vi "TestCloneAPI.vi"() -> ()   [LabVIEW 2014, in "FGenModule.lvlib"]
uses:
  FGenModule.lvlib
  FGenPlugins/MyPluginBaseClass/TypeDef/OperateModeParams.ctl
  FGenPlugins/MyPluginBaseClass/TypeDef/OutputEnableParams.ctl
  FGenPlugins/MyPluginBaseClass/TypeDef/OutputModeParams.ctl
  FGenPlugins/MyPluginBaseClass/TypeDef/RefClkSourceParams.ctl
  FGenPlugins/MyPluginBaseClass/TypeDef/ChannelNameParams.ctl
  FGenPlugins/MyPluginBaseClass/TypeDef/ConfigStdWaveformParams.ctl
  FGenPlugins/MyPluginBaseClass/TypeDef/ClrArbWfrmParams.ctl
  FGenPlugins/MyPluginBaseClass/TypeDef/CreateArbWfrmParams.ctl
  FGenPlugins/MyPluginBaseClass/TypeDef/ConfigArbWfrmParams.ctl
  FGenPlugins/MyPluginBaseClass/TypeDef/ConfigArbWfrmSRatParams.ctl
  FGenPlugins/MyPluginBaseClass/TypeDef/TriggerParams.ctl
  FGenPlugins/MyPluginBaseClass/TypeDef/ChannelParams.ctl
  FGenPlugins/MyPluginBaseClass/TypeDef/ChannelParamElement.ctl
  <userlib>/NIST/ModuleAdminLib/ModuleAdmin/ModuleAdmin.lvclass/ModuleAdmin.ctl
  <userlib>/NIST/ModuleAdminLib/ModuleAdmin/ModuleAdmin.lvclass
  FGenPlugins/MyPluginBaseClass/TypeDef/PluginParams.ctl
  PublicAPI/Arguments/Broadcasts/clDidInit.ctl
  PublicAPI/Arguments/Requests/clStopArgument.ctl
  <userlib>/NIST/ModuleAdminLib/ModuleAdmin/Accessors/Read CloneRegRef.vi
  <userlib>/NIST/ModuleAdminLib/CloneRegistration/CloneRegistration.lvclass
  FGenPlugins/MyPluginBaseClass/NISTFGenPluginsBase.lvclass
panel:
  in  "btnGetTimestamp":bool
  out "Timestamp":timestamp format="%^<%.3X\n%x>T"
  in  "btnConfigDlg":bool
  out "error out":errorcluster
  in  "btnWriteChannel":bool
  in  "btnReadChannel":bool
  in  "ChannelParams":T1 {"eOutputMode" items=["Function", "Arbitrary", "Sequence"]; "eOperateMode" items=["Continuous", "Burst"]}
  in  "btnGetDefaults":bool
  in  "Plugin Type":u16(ring) items=["Keysight 335XX", "none", "HIL FGen", "NI Dynamic 2", "NI Dyn3 FGen", "NI PXI 6733"]
  in  "btnListVISA":bool
  in  "btnSetTrigger":bool
  in  "TriggerParams":T3={"eTrigger"=0, "eEdge"=10280, "sSource"="/PXI1Slot7/PFI1"} {"eEdge" items=["Rising"=10280, "Falling"=10171]; "eTrigger" items=["None", "Digital", "Analog"]}
  in  "ConfigArbWfrmSRatParams":T4
  in  "btnConfigArbWfrmSRat":bool
  in  "ArbWfrmConfig":T5
  in  "btnConfigArbWfrm":bool
  in  "CreateArbWfrmParams":T6={"sName"="1", "iSize"=8, "dData"=[1.0, 1.0, 2.0, 2.5, 2.5, 1.8, 1.8, 1.9, 2.7, 2.9, 1.2], "sWfrmHandle"="ARB1"}
  in  "btnCreateArbWfrm":bool
  in  "ClrArbWfrmParams":T7
  in  "btnClearArbWfrm":bool
  in  "ConfigStdWaveformParams":T8={"sName"="1", "eWaveform"=0, "dAmplitude"=1.0, "dDcOffset"=0.0, "dFrequency"=10.0, "dStartPhase"=0.0, "dSampleRate"=4800.0, "dNumSamples"=4800.0} {"eWaveform" items=["Sine"=0, "Square"=1, "Ramp"=2, "Noise"=3, "DC"=4, "Triangle"=5, "Pulse"=6, "Sinc"=11, "D-Lorentz"=12, "Gaussian"=13, "Expo Fall"=14, "Expo Rise"=15, "Haversine"=16]}
  in  "btnSetStdWaveform":bool
  in  "btnInitialize":bool
  in  "btnReset":bool
  in  "btnAbortGeneration":bool
  out "Channel Name":string
  in  "ChannelNameParams":T9
  in  "RefClkSourceParams":T10 {"eRefClk" items=["Internal", "External", "RTSI"]}
  in  "OutputModeParams":T11 {"eOutputMode" items=["Function", "Arbitrary", "Sequence"]}
  in  "btnInitiateGeneration":bool
  in  "btnChannelNameRequest":bool
  in  "btnSetRefClkSource":bool
  in  "btnSetOutputMode":bool
  in  "OutputEnableParams":T12
  in  "btnSetOutputEnable":bool
  in  "btnSetOperateMode":bool
  in  "OperateModeParams":T13 {"eOperateMode" items=["Continuous", "Burst"]}
  in  "btnLoadPlugin":bool
  out "Path":path
  in  "btnRequestINIPath":bool
  in  "btnRemove":bool
  out "Status Log":string
  out "Active Modules (Array)":string[](array[string])
  in  "btnAdd":bool
  in  "btnStop":bool
  in  "Select Module":i32(ring)=-1 caption="Select Module to send Request" items=["All"=-1]
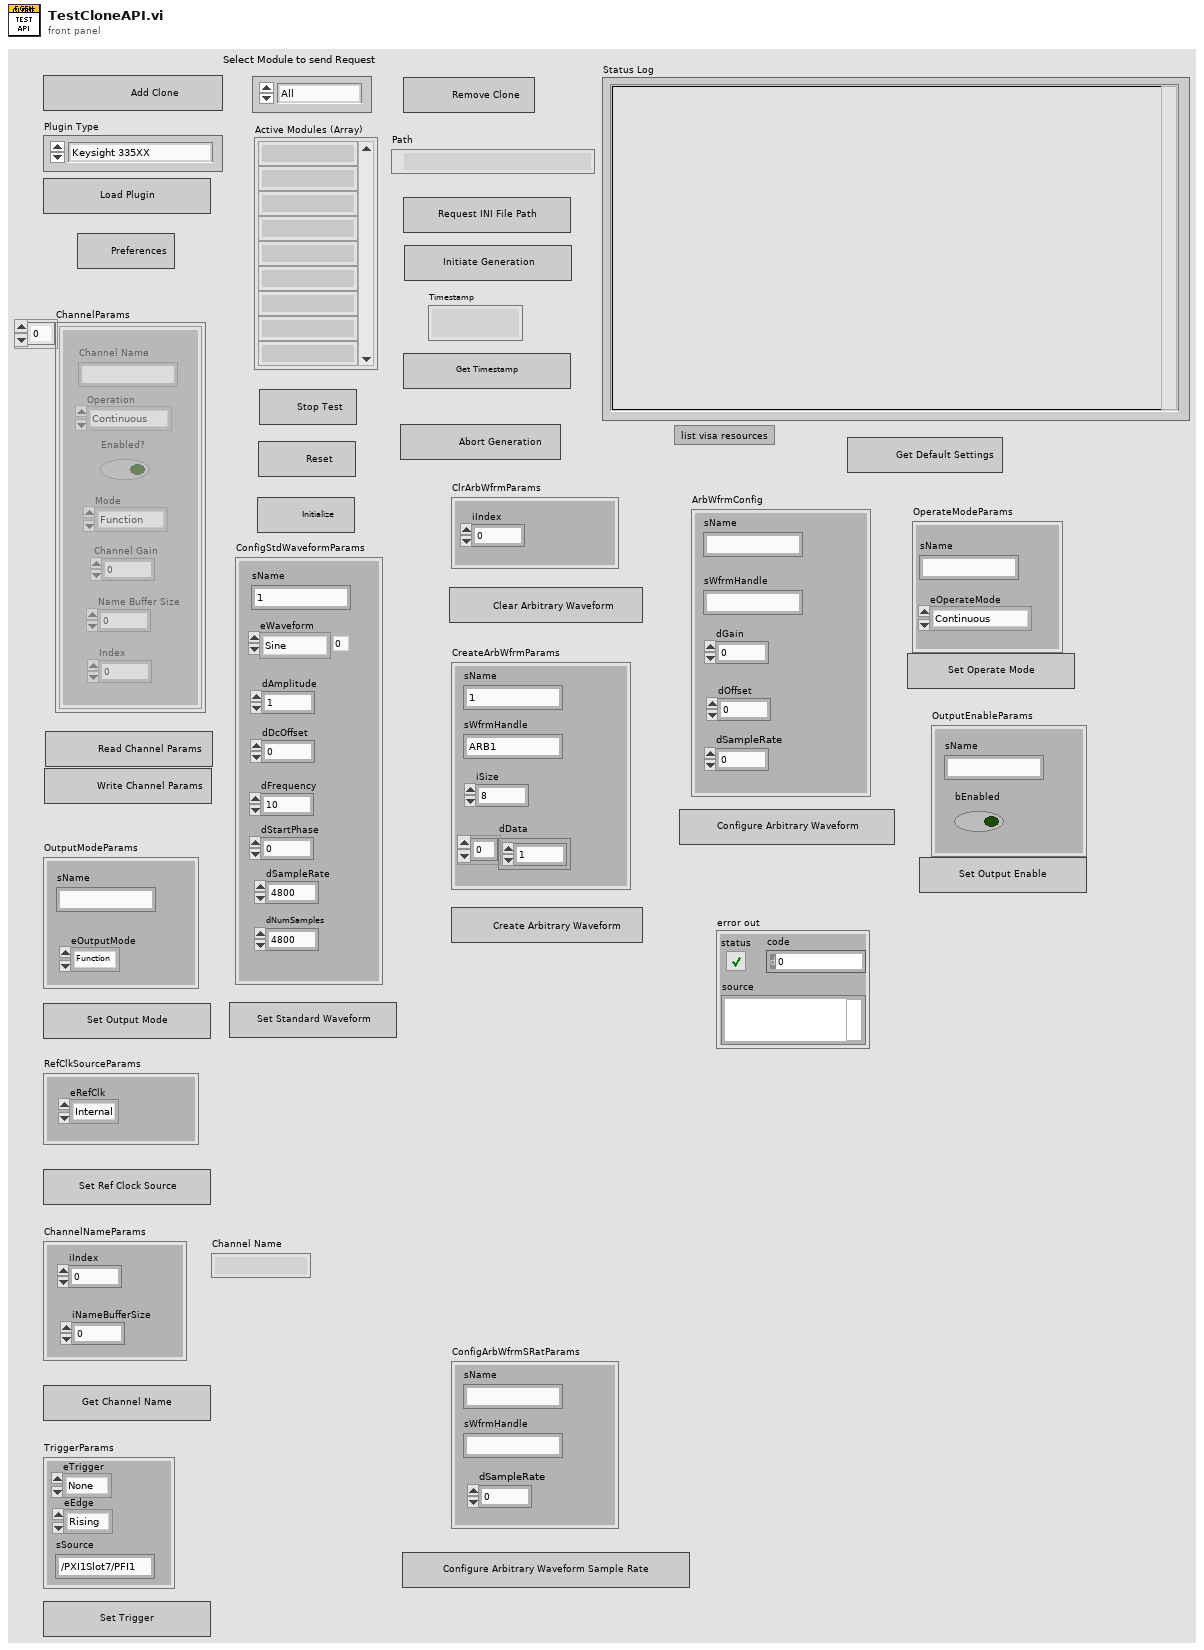
[diagram p1: front panel]
types:
  T1 = typedef "FGenPlugins.lvlib/NISTFGenPluginsBase.lvclass/ChannelParams.ctl" = T2[]
  T2 = typedef "FGenPlugins.lvlib/NISTFGenPluginsBase.lvclass/ChannelParamElement.ctl" = cluster{"sName":string, "eOperateMode":u16, "bEnabled":bool, "eOutputMode":u16, "iIndex":i32, "iNameBufferSize":i32, "fGain":dbl}
  T3 = typedef "FGenPlugins.lvlib/NISTFGenPluginsBase.lvclass/TriggerParams.ctl" = cluster{"eTrigger":u16, "eEdge":u16, "sSource":string}
  T4 = typedef "FGenPlugins.lvlib/NISTFGenPluginsBase.lvclass/ConfigArbWfrmSRatParams.ctl" = cluster{"sName":string, "dSampleRate":dbl, "sWfrmHandle":string}
  T5 = typedef "FGenPlugins.lvlib/NISTFGenPluginsBase.lvclass/ConfigArbWfrmParams.ctl" = cluster{"sName":string, "dGain":dbl, "sWfrmHandle":string, "dOffset":dbl, "dSampleRate":dbl}
  T6 = typedef "FGenPlugins.lvlib/NISTFGenPluginsBase.lvclass/CreateArbWfrmParams.ctl" = cluster{"sName":string, "iSize":i32, "dData":dbl[], "sWfrmHandle":string}
  T7 = typedef "FGenPlugins.lvlib/NISTFGenPluginsBase.lvclass/ClrArbWfrmParams.ctl" = cluster{"iIndex":i32}
  T8 = typedef "FGenPlugins.lvlib/NISTFGenPluginsBase.lvclass/ConfigStdWaveformParams.ctl" = cluster{"sName":string, "eWaveform":u16, "dAmplitude":dbl, "dDcOffset":dbl, "dFrequency":dbl, "dStartPhase":dbl, "dSampleRate":dbl, "dNumSamples":dbl}
  T9 = typedef "FGenPlugins.lvlib/NISTFGenPluginsBase.lvclass/ChannelNameParams.ctl" = cluster{"iIndex":i32, "iNameBufferSize":i32}
  T10 = typedef "FGenPlugins.lvlib/NISTFGenPluginsBase.lvclass/RefClkSourceParams.ctl" = cluster{"eRefClk":u16}
  T11 = typedef "FGenPlugins.lvlib/NISTFGenPluginsBase.lvclass/OutputModeParams.ctl" = cluster{"sName":string, "eOutputMode":u16}
  T12 = typedef "FGenPlugins.lvlib/NISTFGenPluginsBase.lvclass/OutputEnableParams.ctl" = cluster{"sName":string, "bEnabled":bool}
  T13 = typedef "FGenPlugins.lvlib/NISTFGenPluginsBase.lvclass/OperateModeParams.ctl" = cluster{"sName":string, "eOperateMode":u16}
  T14 = typedef "FGenModule.lvlib/clBroadcastEvents.ctl" = cluster{"DidInit":refnum<user-event>, "StatusUpdate":refnum<user-event>, "ErrorReport":refnum<user-event>, "DidStop":refnum<user-event>, "PathToINI":refnum<user-event>, "ChannelName":refnum<user-event>, "ArbWfrmConfig":refnum<user-event>, "ChannelParams":refnum<user-event>, "Timestamp":refnum<user-event>}
  T15 = typedef "FGenPlugins.lvlib/NISTFGenPluginsBase.lvclass/PluginParams.ctl" = cluster{"Path to Plugin INI":path}
  T16 = typedef "FGenModule.lvlib/clDidInit.ctl" = cluster{"Init?":bool, "ModuleAdmin":refnum<class "ModuleAdmin.lvclass">}
  T17 = typedef "FGenModule.lvlib/clStopArgument.ctl" = cluster{"Exit via Stop Module Req?":bool, "Wait for Module to stop?":bool, "ModuleAdmin":refnum<class "ModuleAdmin.lvclass">}
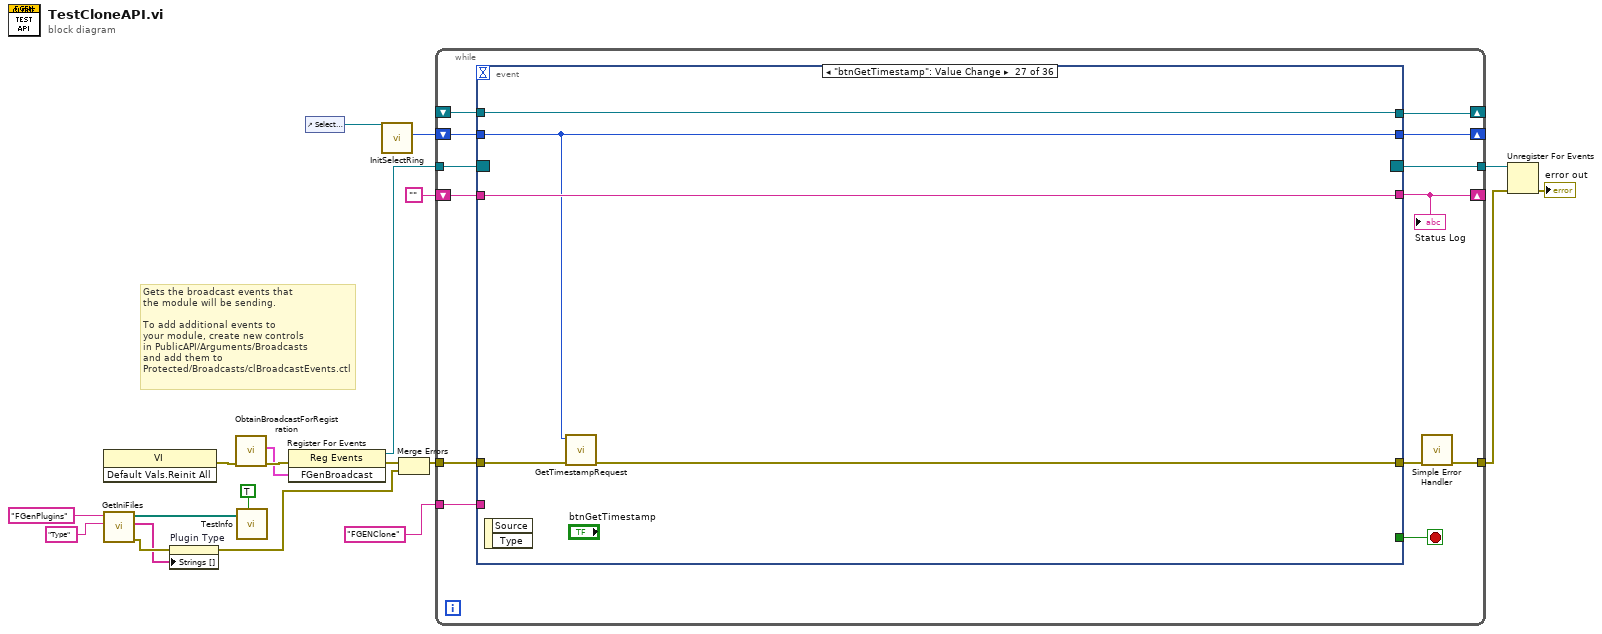
[diagram p0: block diagram]
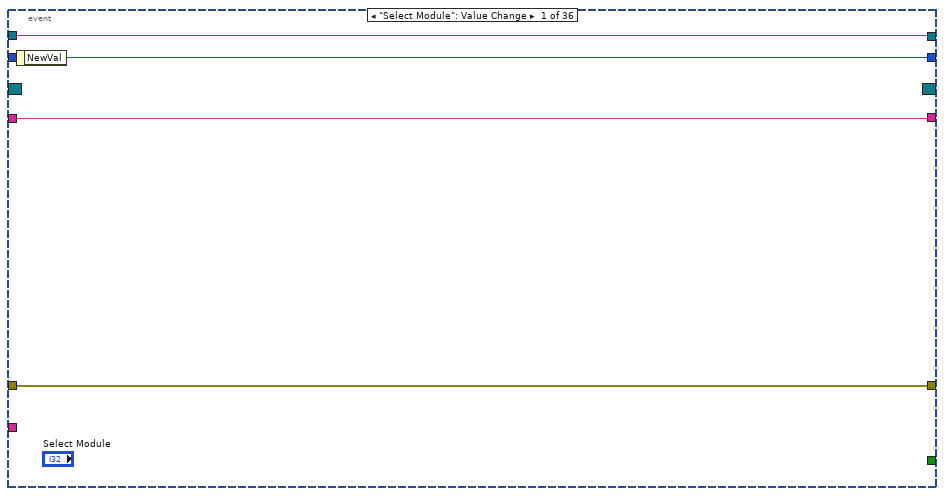
[diagram p2: hidden frame]
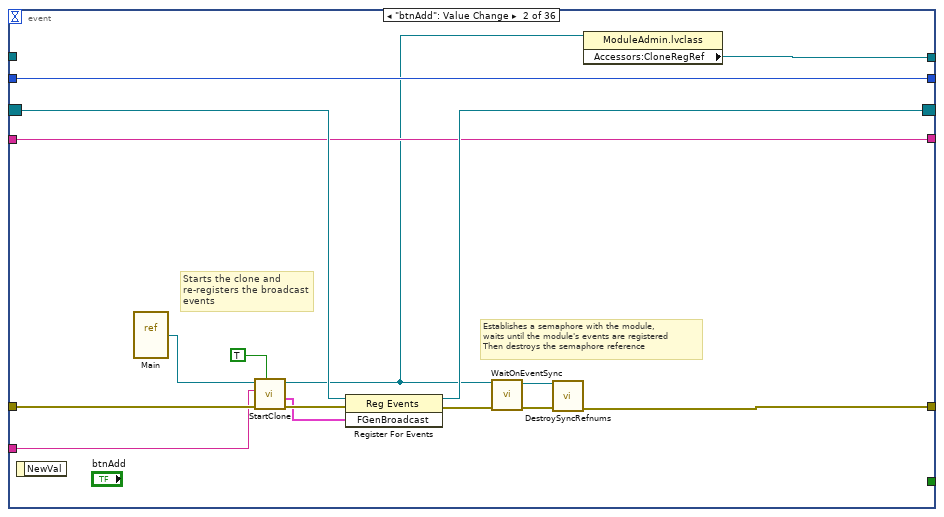
[diagram p3: hidden frame]
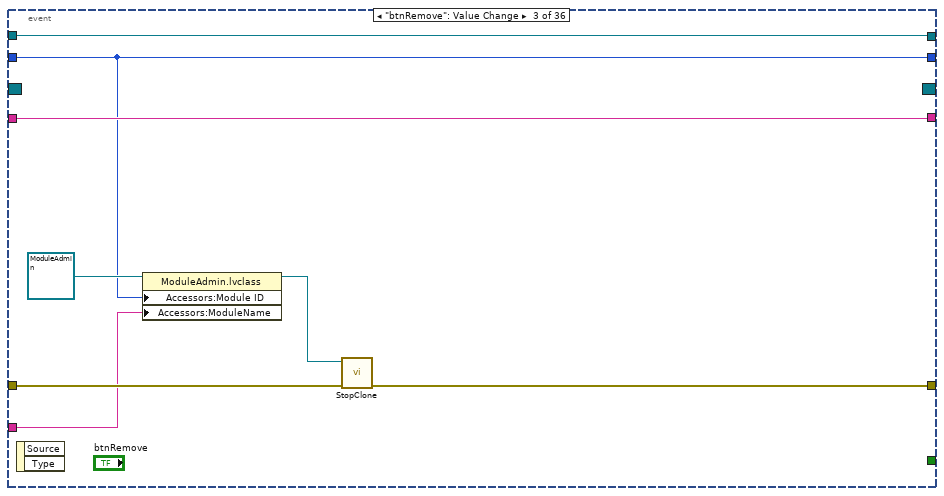
[diagram p4: hidden frame]
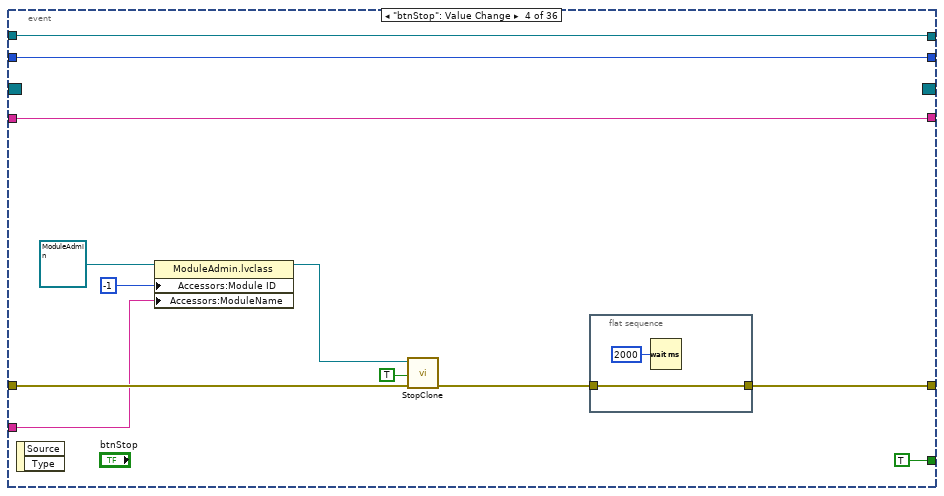
[diagram p5: hidden frame]
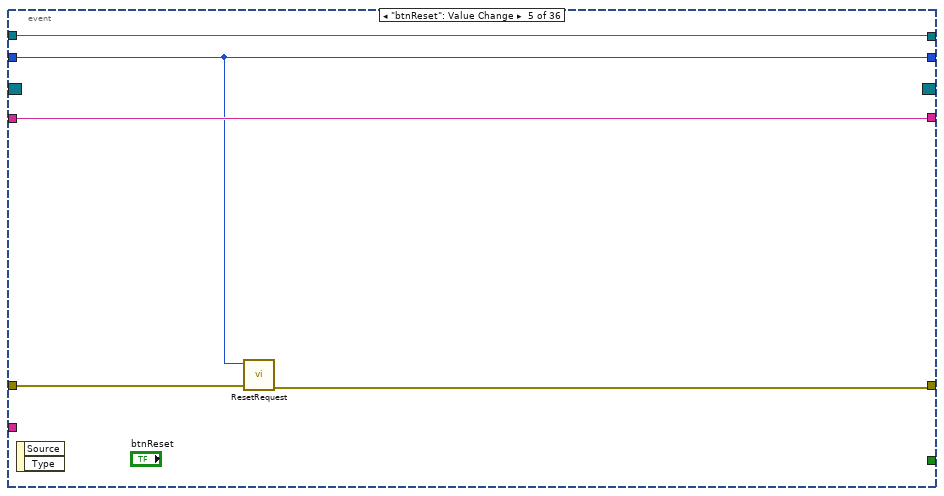
[diagram p6: hidden frame]
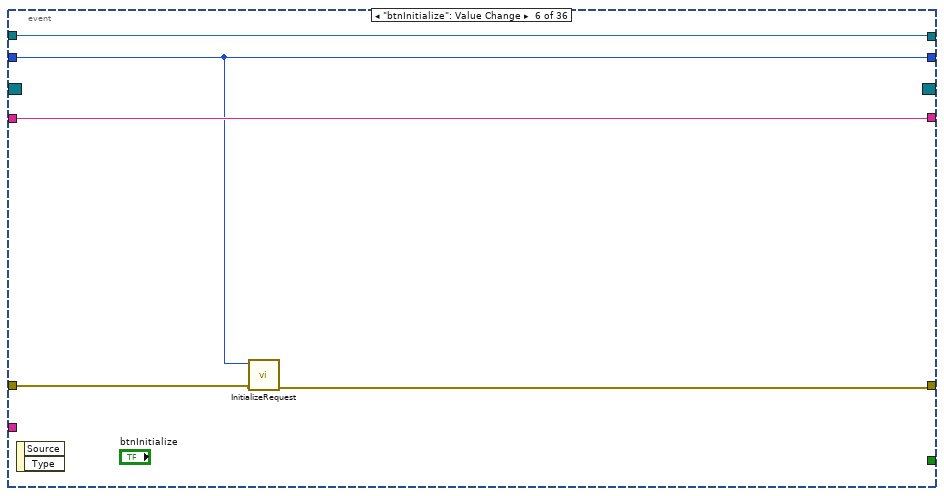
[diagram p7: hidden frame]
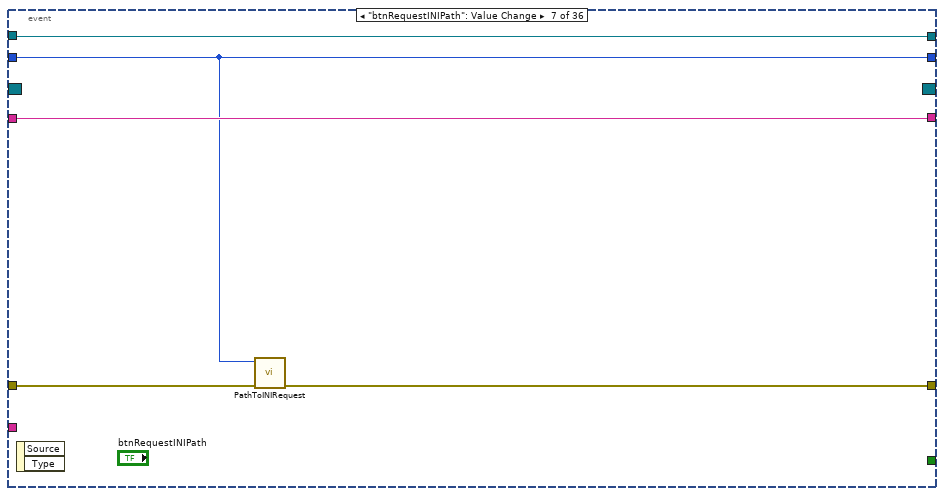
[diagram p8: hidden frame]
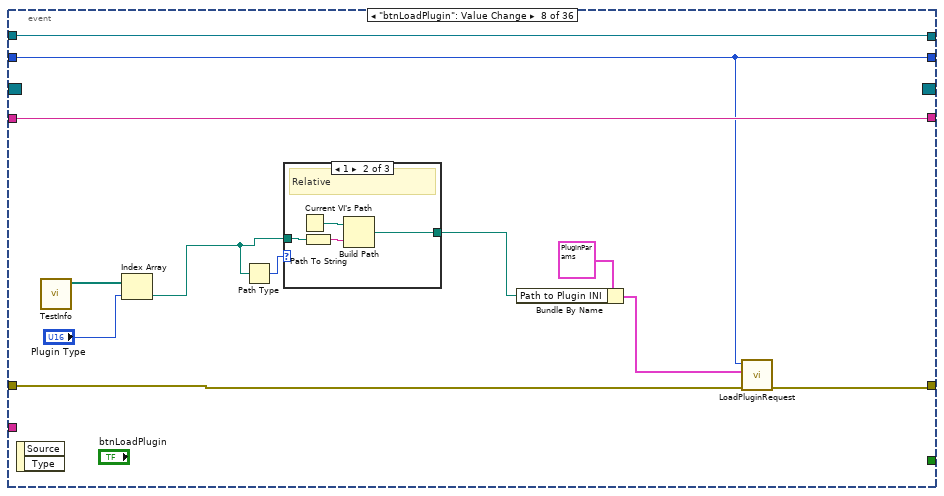
[diagram p9: hidden frame]
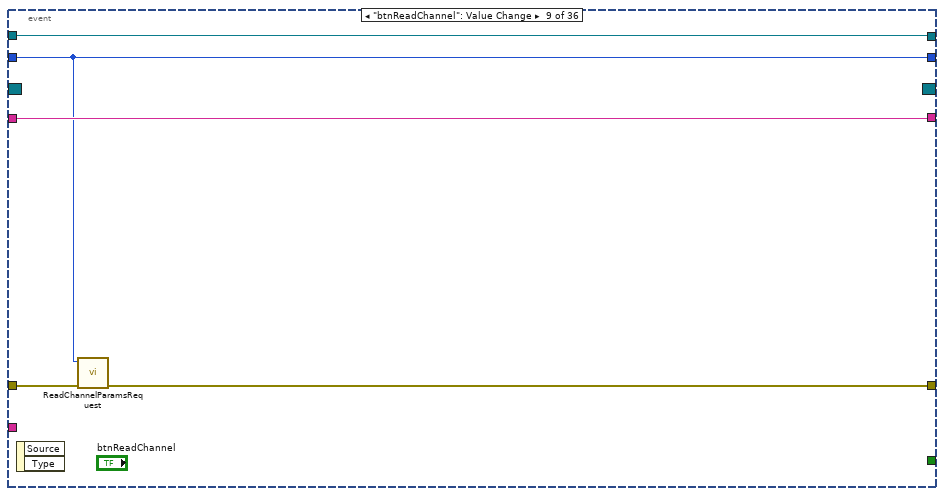
[diagram p12: hidden frame]
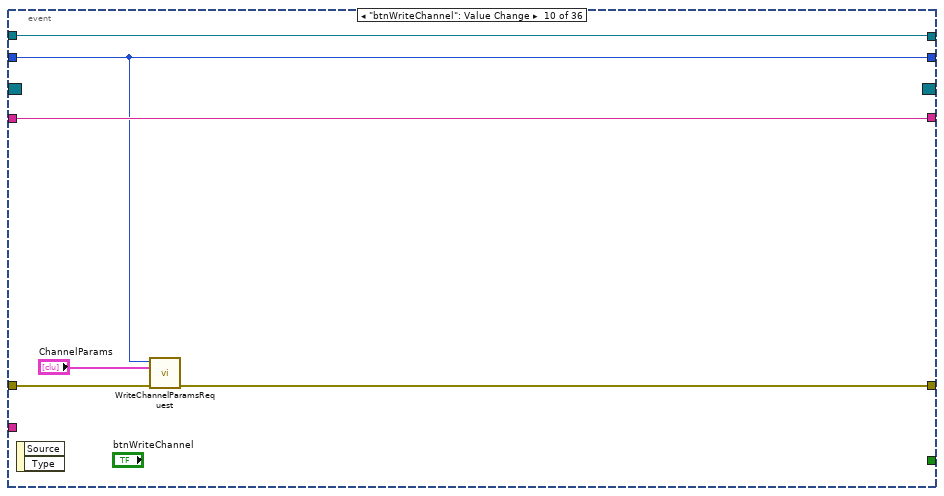
[diagram p13: hidden frame]
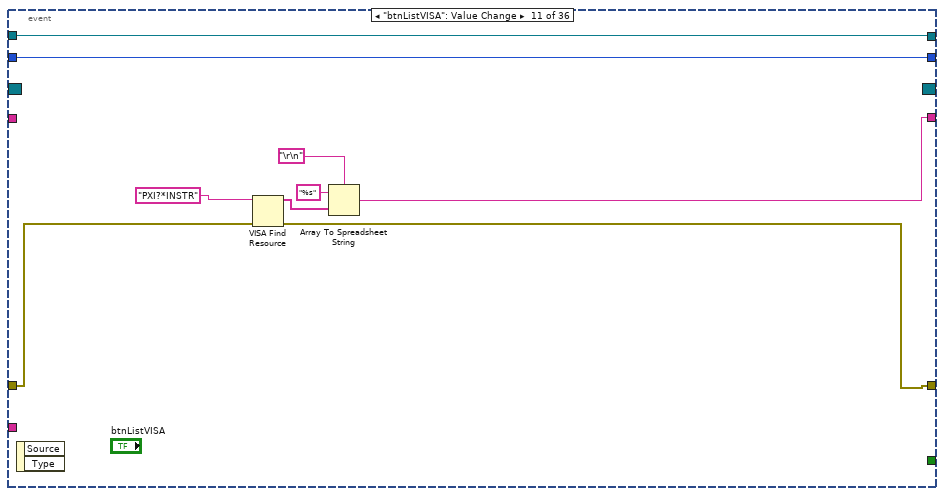
[diagram p14: hidden frame]
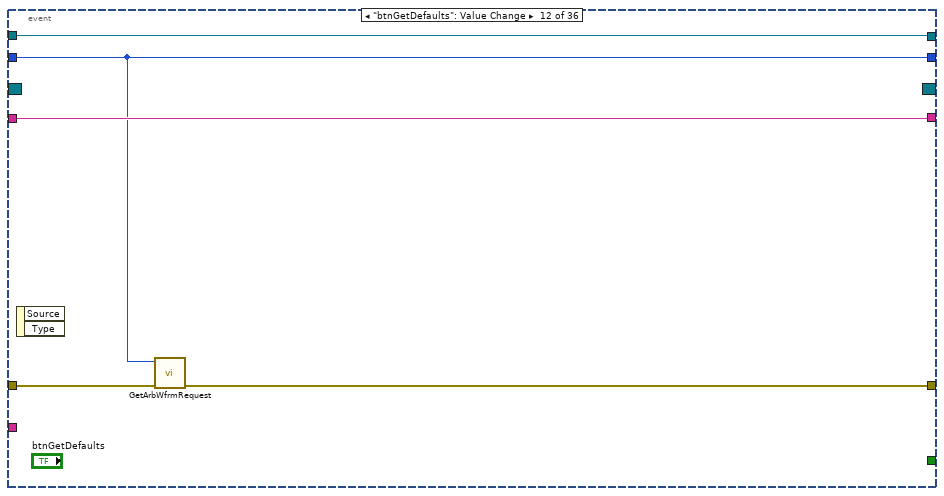
[diagram p15: hidden frame]
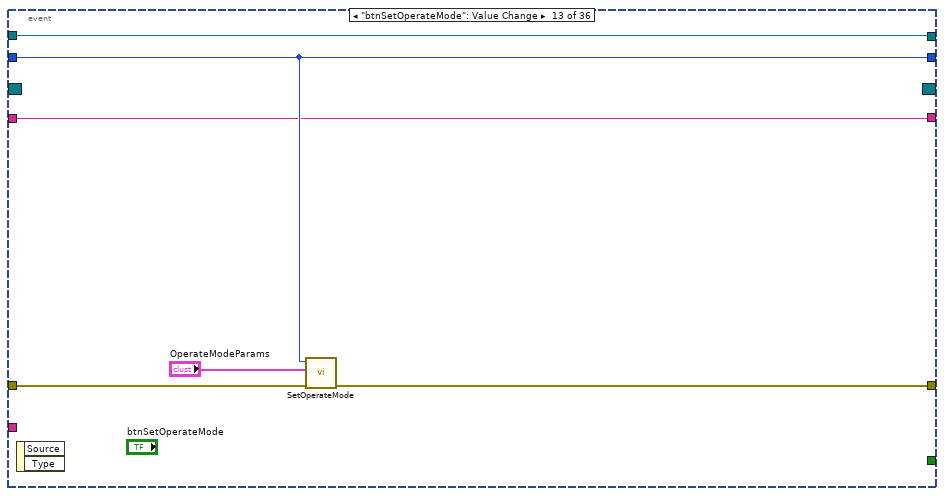
[diagram p16: hidden frame]
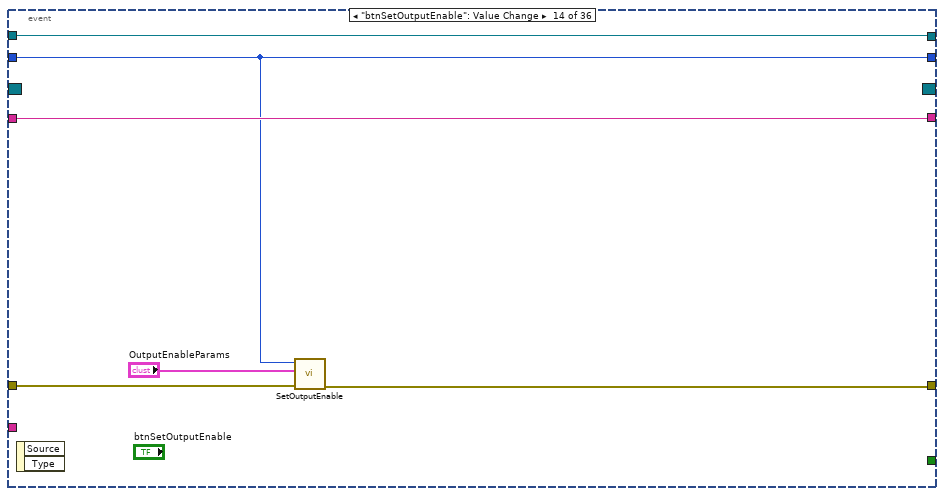
[diagram p17: hidden frame]
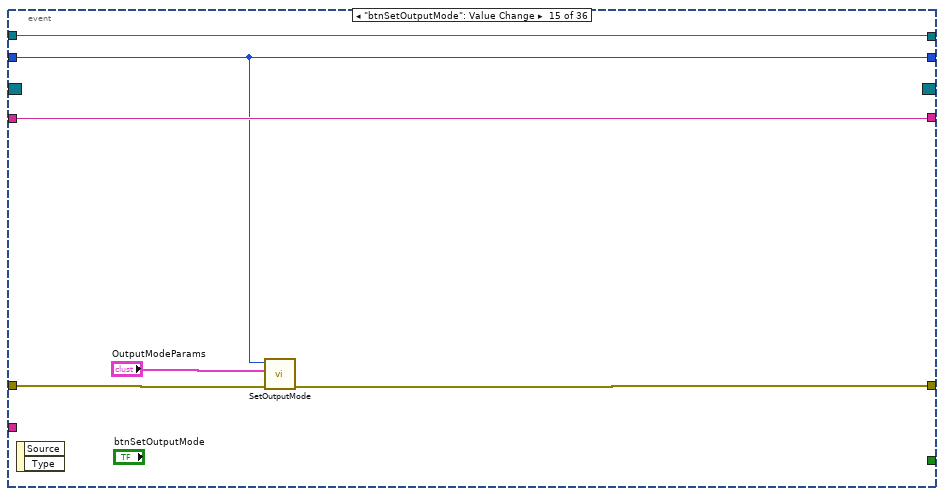
[diagram p18: hidden frame]
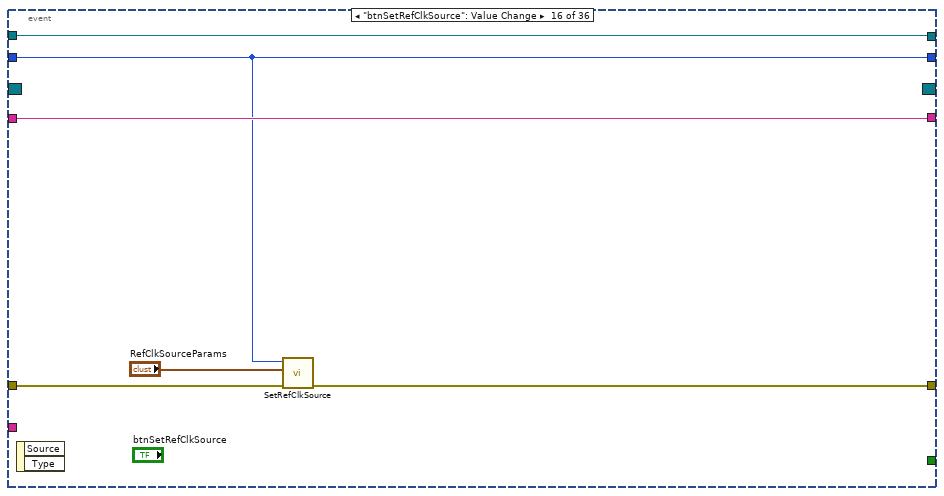
[diagram p19: hidden frame]
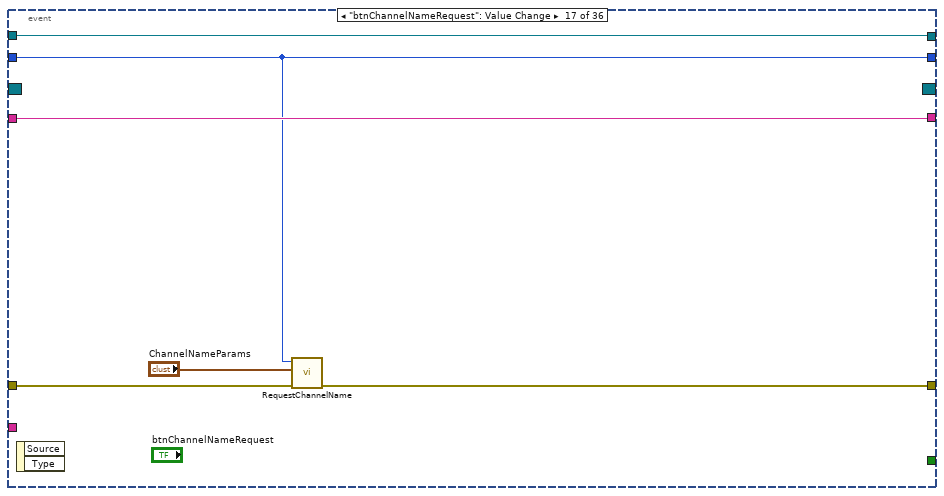
[diagram p20: hidden frame]
diagram:
  # "Gets the broadcast events that\nthe module will be sending.\n\nTo add additional events to\nyour module, create new controls\nin PublicAPI/Arguments/Broadcasts\nand add them to\nProtected/Broadcasts/clBroadcastEvents.ctl"
  n1 = invoke class="VI" method="Default Vals.Reinit All"() -> (error out=w18:errorcluster)  [unwired: 3 in, 2 out]
  n2 = call "GetIniFiles.vi"("iniKey"="Type", "name or relative path"="FGenPlugins") -> ("error out"=w9:errorcluster, "Types"=w4:string[], "IniFilePaths"=w8:path[])  [unwired: 7 in]
  n3 = property on="Plugin Type" class="Ring (strict)"(error in=w9, "Strings []"=w4) -> (error out=w5:errorcluster)  [unwired: 1 in, 1 out]
  n4 = call "ObtainBroadcastForRegistration.vi"("error in (no error)"=w18) -> ("error out"=w17:errorcluster, "FGenBroadcast"=w16:T14)  [unwired: 9 in]
  n5 = call "TestInfo.vi"("Set (f)"=TRUE, "PluginIniFilePaths"=w8) -> ()  [unwired: 9 in, 1 out]
  n6 = register-events(error in=w17, w16) -> (reference out=w14:refnum<event-registration>, error out=w15:errorcluster)  [unwired: 1 in]
  n7 = control-ref of="Select Module"() -> (w20:refnum<vi>)
  n8 = call "InitSelectRing.vi"("Ring Refnum"=w20) -> ("Module Ring Value"=w19:i32)  [unwired: 9 in, 1 out]
  n9 = Merge Errors(w15, w5) -> (w6:errorcluster)
  n10 = while {
    shift-right: [w32] -> _
    shift-left: w19 -> [w33]
    tunnel: w6 -> [w30]
    tunnel: w14 -> [w27]
    tunnel: [w28] -> w2
    shift-right: [w26] -> _
    shift-left: "" -> [w25]
    tunnel: "FGENClone" ("ModuleName") -> [w24]
    tunnel: [w23] -> w3
    shift-right: [w22] -> _
    shift-left: _ -> [w21]
    stop <- w31 stop-if-true
    n11 = event shown="[26] \"btnGetTimestamp\": Value Change" {
      selector: w27 -> [_ w45 _ _ _ _ _ _ _ _ _ _ _ _ _ _ _ _ _ _ _ _ _ _ _ _ _ _ _ _ _ _ _ _ _ _]
      dyn-events: [_ w44 _ _ _ _ _ _ _ _ _ _ _ _ _ _ _ _ _ _ _ _ _ _ _ _ _ _ _ _ _ _ _ _ _ _] -> w23
      timeout: _ -> [_ _ _ _ _ _ _ _ _ _ _ _ _ _ _ _ _ _ _ _ _ _ _ _ _ _ _ _ _ _ _ _ _ _ _ _]
      tunnel: w33 -> [_ w53 w57 w73 w77 w84 w89 w100 w111 w116 w124 w131 w136 w141 w149 w155 w159 w165 w170 w176 w182 w188 w194 w201 w206 w210 w215 _ _ w283 w288 w300 w309 w312 w320 w333]
      tunnel: [w37 w53 w57 w73 w77 w84 w89 w100 w111 w116 w124 w131 w136 w141 w149 w155 w159 w165 w170 w176 w182 w188 w194 w201 w206 w210 w215 w238 w254 w283 w288 w300 w309 w312 w320 w333] -> w32
      tunnel: [_ _ _ TRUE _ _ _ _ _ _ _ _ _ _ _ _ _ _ _ _ _ _ _ _ _ _ _ _ _ _ _ _ _ _ _ _] -> w31
      tunnel: w30 -> [w35 w52 w60 w71 w79 w83 w88 w101 w113 w119 w125 w132 w138 w144 w148 w154 w161 w167 w172 w178 w184 w190 w196 w203 w208 w213 w219 w243 w263 w280 w292 w296 w307 w317 w327 w336]
      tunnel: [w35 w46 w59 w64 w78 w82 w87 w99 w110 w115 w126 w130 w137 w143 w147 w153 w160 w166 w171 w177 w183 w189 w195 w202 w205 w212 w218 w227 w251 w274 w291 w295 w306 w313 w322 w328] -> w29
      tunnel: [w36 w42 w61 w69 w80 w85 w90 w102 w112 w117 w127 w133 w135 w145 w151 w157 w163 w168 w173 w179 w185 w191 w197 w200 w209 w211 w216 w231 w260 w277 w287 w301 w308 w311 w321 w332] -> w26
      tunnel: w25 -> [w36 w42 w61 w69 w80 w85 w90 w102 w112 w117 _ w133 w135 w145 w151 w157 w163 w168 w173 w179 w185 w191 w197 w200 w209 w211 w216 w230 w261 w282 w287 w301 w308 w311 w321 w332]
      tunnel: w24 -> [_ w41 w56 w66 _ _ _ _ _ _ _ _ _ _ _ _ _ _ _ _ _ _ _ _ _ _ _ _ _ _ _ _ _ _ _ _]
      tunnel: [w34 w38 w54 w62 w76 w81 w86 w91 w109 w114 w120 w129 w134 w140 w146 w152 w158 w164 w169 w174 w180 w186 w192 w198 w204 w214 w217 w220 w244 w268 w284 w294 w302 w310 w319 w334] -> w22
      tunnel: w21 -> [w34 _ w54 w62 w76 w81 w86 w91 w109 w114 w120 w129 w134 w140 w146 w152 w158 w164 w169 w174 w180 w186 w192 w198 w204 w214 w217 w220 w244 w268 w284 w294 w302 w310 w319 w334]
      event "Select Module": Value Change {
        n12 = event-data() -> ("NewVal"=w37:i32)  [unwired: 1 in]
      }
      event "btnAdd": Value Change {
        # "Establishes a semaphore with the module,\nwaits until the module's events are registered\nThen destroys the semaphore reference"
        # "Starts the clone and\nre-registers the broadcast \nevents"
        n13 = event-data() -> ()  [unwired: 1 in, 1 out]
        n14 = vi-ref "Main.vi"() -> (w43:refnum<vi>)
        n15 = call "StartClone.vi"("ShowPanel? (F)"=TRUE, "error in (no error)"=w52, "ModuleName"=w41, "VI Refnum"=w43) -> ("error out"=w51:errorcluster, "FGenBroadcast"=w47:T14, "ModuleAdmin"=w39:refnum<class "ModuleAdmin.lvclass">)  [unwired: 5 in]
        n16 = register-events(reference=w45, error in=w51, w47) -> (reference out=w44:refnum<event-registration>, error out=w50:errorcluster)
        n17 = call <userlib>:"WaitOnEventSync.vi"("error in (no error)"=w50, "ModuleAdmin"=w39) -> ("error out"=w49:errorcluster, "ModuleAdmin"=w48:refnum<class "ModuleAdmin.lvclass">)  [unwired: 8 in]
        n18 = call <userlib>:"DestroySyncRefnums.vi"("error in (no error)"=w49, "ModuleAdmin"=w48) -> ("error out"=w46:errorcluster)  [unwired: 9 in]
        n19 = property class="ModuleAdmin.lvclass"(reference=w39) -> ("Accessors:CloneRegRef"=w38:refnum<data-value>)  [unwired: 1 in, 2 out]
      }
      event "btnRemove": Value Change {
        n20 = event-data() -> ()  [unwired: 1 in, 2 out]
        n21 = property class="ModuleAdmin.lvclass"(reference=refnum<class "ModuleAdmin.lvclass"> refnum ("ModuleAdmin.lvlib:ModuleAdmin.lvclass"), "Accessors:Module ID"=w57, "Accessors:ModuleName"=w56) -> (reference out=w55:refnum<class "ModuleAdmin.lvclass">)  [unwired: 1 in, 1 out]
        n22 = call "StopClone.vi"("error in (no error)"=w60, "ModuleAdmin"=w55) -> ("error out"=w59:errorcluster)  [unwired: 9 in]
      }
      event "btnStop": Value Change {
        n23 = event-data() -> ()  [unwired: 1 in, 2 out]
        n24 = property class="ModuleAdmin.lvclass"(reference=refnum<class "ModuleAdmin.lvclass"> refnum ("ModuleAdmin.lvlib:ModuleAdmin.lvclass"), "Accessors:Module ID"=-1 ("Module ID"), "Accessors:ModuleName"=w66) -> (reference out=w65:refnum<class "ModuleAdmin.lvclass">)  [unwired: 1 in, 1 out]
        n25 = call "StopClone.vi"("error in (no error)"=w71, "Wait for Module to stop?"=TRUE, "ModuleAdmin"=w65) -> ("error out"=w63:errorcluster)  [unwired: 8 in]
        n26 = flat-sequence {
          tunnel: [w74] -> w64
          tunnel: w63 -> [w74]
          frame #0 {
            n27 = Wait (ms)(milliseconds to wait=u32 2000) -> ()  [unwired: 1 out]
          }
        }
      }
      event "btnReset": Value Change {
        n28 = event-data() -> ()  [unwired: 1 in, 2 out]
        n29 = call "ResetRequest.vi"("error in (no error)"=w79, "ModuleID"=w77) -> ("error out"=w78:errorcluster)  [unwired: 9 in]
      }
      event "btnInitialize": Value Change {
        n30 = event-data() -> ()  [unwired: 1 in, 2 out]
        n31 = call "InitializeRequest.vi"("error in (no error)"=w83, "ModuleID"=w84) -> ("error out"=w82:errorcluster)  [unwired: 9 in]
      }
      event "btnRequestINIPath": Value Change {
        n32 = event-data() -> ()  [unwired: 1 in, 2 out]
        n33 = call "PathToINIRequest.vi"("error in (no error)"=w88, "ModuleID"=w89) -> ("error out"=w87:errorcluster)  [unwired: 9 in]
      }
      event "btnLoadPlugin": Value Change {
        n34 = event-data() -> ()  [unwired: 1 in, 2 out]
        n35 = call "TestInfo.vi"() -> ("PluginIniFilePaths"=w95:path[])  [unwired: 11 in]
        n36 = Index Array(array=w95, index="Plugin Type") -> (element=w93:path)
        n37 = Path Type(1:w93) -> (0:w98:i16)
        n38 = case shown="1" w98 {
          tunnel: w93 -> [w103 w105 w108]
          tunnel: [w103 w104 w108] -> w96
          frame 0, Default {
            # "Absolute"
          }
          frame 1 {
            # "Relative"
            n39 = Current VI's Path() -> (path=w106:path)
            n40 = Path To String(path=w105) -> (string=w107:string)
            n41 = Build Path(base path=w106, name or relative path=w107) -> (appended path=w104:path)
          }
          frame 2 {
            # "Not a Path"
          }
        }
        n42 = Bundle By Name(cluster=T15 {"Path to Plugin INI"=path "../../FGenPlugins/NiPxi6733/NiPxi6733.ini"} ("PluginParams"), "Path to Plugin INI"=w96) -> (w97:T15)
        n43 = call "LoadPluginRequest.vi"("error in (no error)"=w101, "PluginParams"=w97, "ModuleID"=w100) -> ("error out"=w99:errorcluster)  [unwired: 8 in]
      }
      event "btnReadChannel": Value Change {
        n44 = event-data() -> ()  [unwired: 1 in, 2 out]
        n45 = call "ReadChannelParamsRequest.vi"("error in (no error)"=w113, "ModuleID"=w111) -> ("error out"=w110:errorcluster)  [unwired: 9 in]
      }
      event "btnWriteChannel": Value Change {
        n46 = event-data() -> ()  [unwired: 1 in, 2 out]
        n47 = call "WriteChannelParamsRequest.vi"("error in (no error)"=w119, "ChannelParams"="ChannelParams", "ModuleID"=w116) -> ("error out"=w115:errorcluster)  [unwired: 8 in]
      }
      event "btnListVISA": Value Change {
        n48 = event-data() -> ()  [unwired: 1 in, 2 out]
        n49 = VISA Find Resource(8:w125, 11:"PXI?*INSTR" ("expression (\"?*\")")) -> (0:w126:errorcluster, 3:w122:string[])  [unwired: 1 in, 1 out]
        n50 = Array To Spreadsheet String(delimiter (Tab)="\r\n", array=w122, 3:"%s" ("format string")) -> (spreadsheet string=w127:string)
      }
      event "btnGetDefaults": Value Change {
        n51 = event-data() -> ()  [unwired: 1 in, 2 out]
        n52 = call "GetArbWfrmRequest.vi"("error in (no error)"=w132, "ModuleID"=w131) -> ("error out"=w130:errorcluster)  [unwired: 9 in]
      }
      event "btnSetOperateMode": Value Change {
        n53 = event-data() -> ()  [unwired: 1 in, 2 out]
        n54 = call "SetOperateMode.vi"("error in (no error)"=w138, "OperateModeParams"="OperateModeParams", "ModuleID"=w136) -> ("error out"=w137:errorcluster)  [unwired: 8 in]
      }
      event "btnSetOutputEnable": Value Change {
        n55 = event-data() -> ()  [unwired: 1 in, 2 out]
        n56 = call "SetOutputEnable.vi"("error in (no error)"=w144, "OutputEnableParams"="OutputEnableParams", "ModuleID"=w141) -> ("error out"=w143:errorcluster)  [unwired: 8 in]
      }
      event "btnSetOutputMode": Value Change {
        n57 = event-data() -> ()  [unwired: 1 in, 2 out]
        n58 = call "SetOutputMode.vi"("error in (no error)"=w148, "OutputModeParams"="OutputModeParams", "ModuleID"=w149) -> ("error out"=w147:errorcluster)  [unwired: 8 in]
      }
      event "btnSetRefClkSource": Value Change {
        n59 = event-data() -> ()  [unwired: 1 in, 2 out]
        n60 = call "SetRefClkSource.vi"("error in (no error)"=w154, "RefClkSourceParams"="RefClkSourceParams", "ModuleID"=w155) -> ("error out"=w153:errorcluster)  [unwired: 8 in]
      }
      event "btnChannelNameRequest": Value Change {
        n61 = event-data() -> ()  [unwired: 1 in, 2 out]
        n62 = call "RequestChannelName.vi"("error in (no error)"=w161, "ChannelNameParams"="ChannelNameParams", "ModuleID"=w159) -> ("error out"=w160:errorcluster)  [unwired: 8 in]
      }
      event "btnInitiateGeneration": Value Change {
        n63 = event-data() -> ()  [unwired: 1 in, 2 out]
        n64 = call "InitiateGenerationRequest.vi"("error in (no error)"=w167, "ModuleID"=w165) -> ("error out"=w166:errorcluster)  [unwired: 9 in]
      }
      event "btnAbortGeneration": Value Change {
        n65 = event-data() -> ()  [unwired: 1 in, 2 out]
        n66 = call "AbortGenerationRequest.vi"("error in (no error)"=w172, "ModuleID"=w170) -> ("error out"=w171:errorcluster)  [unwired: 9 in]
      }
      event "btnSetStdWaveform": Value Change {
        n67 = event-data() -> ()  [unwired: 1 in, 2 out]
        n68 = call "SetStdWaveform.vi"("error in (no error)"=w178, "StdWaveformParams"="ConfigStdWaveformParams", "ModuleID"=w176) -> ("error out"=w177:errorcluster)  [unwired: 8 in]
      }
      event "btnClearArbWfrm": Value Change {
        n69 = event-data() -> ()  [unwired: 1 in, 2 out]
        n70 = call "ClearArbWfrmRequest.vi"("error in (no error)"=w184, "ClrArbWfrmParams"="ClrArbWfrmParams", "ModuleID"=w182) -> ("error out"=w183:errorcluster)  [unwired: 8 in]
      }
      event "btnCreateArbWfrm": Value Change {
        n71 = event-data() -> ()  [unwired: 1 in, 2 out]
        n72 = call "CreateArbWfrmRequest.vi"("error in (no error)"=w190, "CreateArbWfrmParams"="CreateArbWfrmParams", "ModuleID"=w188) -> ("error out"=w189:errorcluster)  [unwired: 8 in]
      }
      event "btnConfigArbWfrm": Value Change {
        n73 = event-data() -> ()  [unwired: 1 in, 2 out]
        n74 = call "ConfigArbWfrmRequest.vi"("error in (no error)"=w196, "ConfigArbWfrmParams"="ArbWfrmConfig", "ModuleID"=w194) -> ("error out"=w195:errorcluster)  [unwired: 8 in]
      }
      event "btnConfigArbWfrmSRat": Value Change {
        n75 = event-data() -> ()  [unwired: 1 in, 2 out]
        n76 = call "ConfigArbWfrmSRatRequest.vi"("error in (no error)"=w203, "ConfigArbWfrmSRatParams"="ConfigArbWfrmSRatParams", "ModuleID"=w201) -> ("error out"=w202:errorcluster)  [unwired: 8 in]
      }
      event "btnSetTrigger": Value Change {
        n77 = event-data() -> ()  [unwired: 1 in, 2 out]
        n78 = call "ConfigTriggerRequest.vi"("error in (no error)"=w208, "TriggerParams"="TriggerParams", "ModuleID"=w206) -> ("error out"=w205:errorcluster)  [unwired: 8 in]
      }
      event "btnConfigDlg": Value Change {
        n79 = event-data() -> ()  [unwired: 1 in, 2 out]
        n80 = call "ConfigureDialogRequest.vi"("error in (no error)"=w213, "ModuleID"=w210) -> ("error out"=w212:errorcluster)  [unwired: 9 in]
      }
      event "btnGetTimestamp": Value Change {
        n81 = event-data() -> ()  [unwired: 1 in, 2 out]
        n82 = call "GetTimestampRequest.vi"("error in (no error)"=w219, "ModuleID"=w215) -> ("error out"=w218:errorcluster)  [unwired: 9 in]
      }
      event User Event {
        # "Adds the module ID to the \nSelect Module ring"
        # "Time stamp and add the DidInit message to the log"
        # "The data types for the broadcast messages\nare in PublicAPI/Broadcasts"
        n83 = event-data() -> ("Data"=w242:variant)  [unwired: 1 in]
        n84 = Variant To Data(error in=w243, type=T16 {"Init?"=FALSE, "ModuleAdmin"=refnum} ("clDidInit"), Variant=w242) -> (data=w235:T16, error out=w240:errorcluster)
        n85 = Unbundle By Name(w235) -> ("ModuleAdmin"=w225:refnum<class "ModuleAdmin.lvclass">)
        n86 = Get Date/Time In Seconds() -> (seconds since 1Jan1904=w233:timestamp)
        n87 = property class="ModuleAdmin.lvclass"(reference=w225) -> ("Accessors:ModuleName"=w223:string, "Accessors:Module ID"=w222:i32, "Accessors:CloneRegRef"=w221:refnum<data-value>)  [unwired: 1 in, 2 out]
        n88 = Get Date/Time String(date format (0)=enum16{"short", "long", "abbreviated"}."short", seconds (now)=w233, want seconds? (F)=TRUE) -> (time string=w236:string)  [unwired: 1 out]
        n89 = Format Into String(format string="%s: %s:%d %s \\r", initial string=w230, w236, w223, w222, "Did Init.") -> (resulting string=w231:string, error out=w228:errorcluster)  [unwired: 1 in]
        n90 = control-ref of="Select Module"() -> (w239:refnum<vi>)
        n91 = call "UpdateSelectRing.vi"("error in (no error)"=w240, "CloneRegRef"=w221, "Ring Refnum"=w239) -> ("error out"=w229:errorcluster, "ActiveModules"=→"Active Modules (Array)":string[], "Module Ring Value"=w238:i32)  [unwired: 6 in]
        n92 = Merge Errors(w229, w228) -> (w227:errorcluster)
      }
      event User Event {
        # "Time stamp and add the Stop message to the log"
        # "The Stop Argument  is found in\nPublicAPI/Arguments/Requests"
        n93 = event-data() -> ("Data"=w262:variant)  [unwired: 1 in]
        n94 = Variant To Data(error in=w263, type=T17 {"Exit via Stop Module Req?"=FALSE, "Wait for Module to stop?"=FALSE, "ModuleAdmin"=refnum} ("Stop Argument"), Variant=w262) -> (data=w258:T17, error out=w257:errorcluster)
        n95 = Unbundle By Name(w258) -> ("ModuleAdmin"=w249:refnum<class "ModuleAdmin.lvclass">)
        n96 = property class="ModuleAdmin.lvclass"(reference=w249) -> ("Accessors:ModuleName"=w247:string, "Accessors:Module ID"=w246:i32, "Accessors:CloneRegRef"=w245:refnum<data-value>)  [unwired: 1 in, 2 out]
        n97 = Get Date/Time In Seconds() -> (seconds since 1Jan1904=w265:timestamp)
        n98 = Get Date/Time String(date format (0)=enum16{"short", "long", "abbreviated"}."short", seconds (now)=w265, want seconds? (F)=TRUE) -> (time string=w267:string)  [unwired: 1 out]
        n99 = Format Into String(format string="%s: %s:%d %s \\r", initial string=w261, w267, w247, w246, "Stopping") -> (resulting string=w260:string, error out=w252:errorcluster)  [unwired: 1 in]
        n100 = control-ref of="Select Module"() -> (w256:refnum<vi>)
        n101 = call "UpdateSelectRing.vi"("error in (no error)"=w257, "CloneRegRef"=w245, "Ring Refnum"=w256) -> ("error out"=w253:errorcluster, "ActiveModules"=w255:string[], "Module Ring Value"=w254:i32)  [unwired: 6 in]
        n102 = local write "Active Modules (Array)"(w255) -> ()
        n103 = Merge Errors(w253, w252) -> (w251:errorcluster)
      }
      event User Event {
        # "Time stamp and add the Status message to the log"
        n104 = event-data() -> ("Data"=w279:variant)  [unwired: 1 in]
        n105 = Variant To Data(error in=w280, type="", Variant=w279) -> (data=w269:string, error out=w276:errorcluster)
        n106 = Get Date/Time In Seconds() -> (seconds since 1Jan1904=w278:timestamp)
        n107 = Get Date/Time String(date format (0)=enum16{"short", "long", "abbreviated"}."short", seconds (now)=w278, want seconds? (F)=TRUE) -> (time string=w271:string)  [unwired: 1 out]
        n108 = Format Into String(format string="%s: %s \\r", initial string=w282, w271, w269) -> (resulting string=w277:string, error out=w275:errorcluster)  [unwired: 1 in]
        n109 = Merge Errors(w276, w275) -> (w274:errorcluster)
      }
      event User Event {
        # "#CodeNeeded\nThis is a very crude error handler\nA better error handler will be needed"
        n110 = event-data() -> ("ModuleID"=w290:i32, "Data"=w293:variant)  [unwired: 1 in]
        n111 = Variant To Data(error in=w292, type=errorcluster {"status"=FALSE, "code"=0, "source"=""} ("error constant"), Variant=w293) -> (data=w286:errorcluster, error out=w291:errorcluster)
        n112 = Number To Decimal String(number=w290) -> (decimal integer string=w289:string)  [unwired: 1 in]
        n113 = call <vilib>:"General Error Handler.vi"("[error source] (\" \")"=w289, "error in (no error)"=w286) -> ()  [unwired: 9 in, 5 out]
      }
      event User Event {
        n114 = event-data() -> ("Data"=w298:variant)  [unwired: 1 in, 1 out]
        n115 = Variant To Data(error in=w296, type=path "" ("Path"), Variant=w298) -> (data=→"Path":path, error out=w295:errorcluster)
      }
      event User Event {
        n116 = event-data() -> ("Data"=w305:variant)  [unwired: 1 in, 1 out]
        n117 = Variant To Data(error in=w307, type="", Variant=w305) -> (data=→"Channel Name":string, error out=w306:errorcluster)
      }
      event User Event {
        n118 = event-data() -> ("Data"=w318:variant)  [unwired: 1 in, 1 out]
        n119 = Variant To Data(error in=w317, type=T5 {"sName"="", "dGain"=0.0, "sWfrmHandle"="", "dOffset"=0.0, "dSampleRate"=0.0} ("ArbWfrmConfig"), Variant=w318) -> (data=w315:T5, error out=w314:errorcluster)
        n120 = property on="ArbWfrmConfig" class="Clust (strict)"(error in=w314, "Value"=w315) -> (error out=w313:errorcluster)  [unwired: 1 in, 1 out]
      }
      event User Event {
        n121 = event-data() -> ("Data"=w326:variant)  [unwired: 1 in, 1 out]
        n122 = Variant To Data(error in=w327, type=T1 [] ("ChannelParams"), Variant=w326) -> (data=w323:T1, error out=w324:errorcluster)
        n123 = property on="ChannelParams" class="Arr (strict)"(error in=w324, "Value"=w323) -> (error out=w322:errorcluster)  [unwired: 1 in, 1 out]
      }
      event User Event {
        n124 = event-data() -> ("Data"=w335:variant)  [unwired: 1 in]
        n125 = Variant To Data(error in=w336, type=0.0, Variant=w335) -> (data=w330:dbl, error out=w328:errorcluster)
        n126 = To Time Stamp(1:w330) -> (0:→"Timestamp":timestamp)
      }
    }
    "Status Log" <- w26
    n127 = call <vilib>:"Simple Error Handler.vi"("error in (no error)"=w29) -> ("error out"=w28:errorcluster)  [unwired: 4 in, 4 out]
  }
  n128 = Unregister For Events(event registration refnum=w3, error in=w2) -> (error out=→"error out":errorcluster)
